vi "Write template.vi"() -> ()   [LabVIEW 2012]
doc: "This VI shows how to use Network Streams to send data."
uses:
  Datatype A.ctl
panel:
  in  "stop":bool
  out "Data A to write":T1
  # "Open \n     Read write template.vi\nfor instructions on how to use this template."
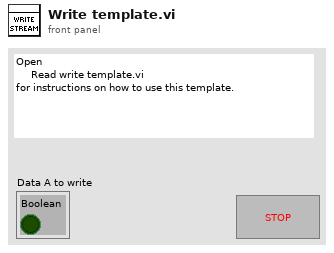
[diagram p1: front panel]
types:
  T1 = typedef "Datatype A.ctl" = cluster{"Boolean":bool}
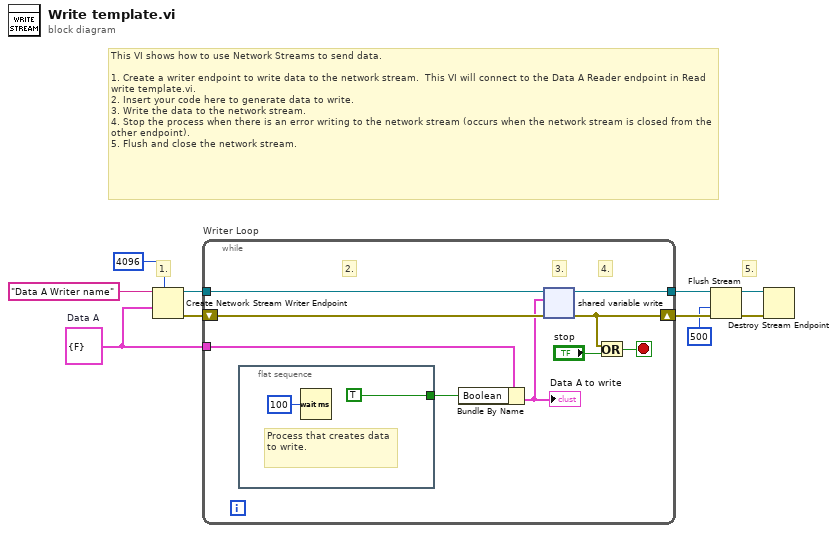
[diagram p0: block diagram]
diagram:
  w9 = T1 {"Boolean"=FALSE}  # Data A
  # "5."
  # "1."
  # "This VI shows how to use Network Streams to send data.\n\n1. Create a writer endpoint to write data to the network stream.  This VI will connect to the Data A Reader endpoint in Read write template.vi.\n2. Insert your code here to generate data to write.\n3. Write the data to the network stream.\n4. Stop the process when there is an error writing to the network stream (occurs when the network stream is closed from the other endpoint).\n5. Flush and close the network stream."
  n1 = Create Network Stream Writer Endpoint(7:4096 ("writer buffer size"), 9:w9, 11:"Data A Writer name" ("writer name")) -> (0:w7:errorcluster, 3:w8:refnum<k21>)  [unwired: 4 in]
  n2 = while "Writer Loop" {
    tunnel: w9 -> [w16]
    tunnel: w8 -> [w19]
    tunnel: [w18] -> w2
    shift-right: [w12] -> w6
    shift-left: w7 -> [w17]
    stop <- w11 stop-if-true
    # "4."
    # "3."
    # "2."
    n3 = flat-sequence {
      tunnel: [TRUE] -> w14
      frame #0 {
        # "Process that creates data to write."
        n4 = Wait (ms)(milliseconds to wait=u32 100) -> ()  [unwired: 1 out]
      }
    }
    n5 = Bundle By Name(cluster=w16, "Boolean"=w14) -> (w15:T1)
    "Data A to write" <- w15
    n6 = shared-variable-write(w19, w17, w15) -> (w18:refnum<k21>, w12:errorcluster)  [unwired: 1 in, 1 out]
    n7 = Or(x=w12, y="stop") -> (x .or. y?=w11:bool)
  }
  n8 = Flush Stream(8:w6, 9:500 ("timeout in ms (-1)"), 11:w2) -> (0:w4:errorcluster, 3:w5:refnum<k21>)  [unwired: 1 in, 1 out]
  n9 = Destroy Stream Endpoint(8:w4, 11:w5) -> ()  [unwired: 1 out]
